vi "smu-dmm-test2.vi"() -> ()   [LabVIEW 2020]
uses:
  Realization/NI DMM/NI DMM.lvclass
  Realization/NI DMM/TypeDefs/DMM waveform settings.ctl
  <instrlib>/niDMM/nidmm.llb/niDMM Waveform Function.ctl
  Realization/NI DMM/TypeDefs/Trigger settings.ctl
  <instrlib>/niDMM/nidmm.llb/niDMM Trigger.ctl
  <instrlib>/niDMM/nidmm.llb/niDMM Slope.ctl
  Realization/PIPX40 Relay/PIPX40 Relay.lvclass
  Realization/PIPX40 Matrix/PIPX40 Matrix.lvclass
  <instrlib>/niDCPower/nidcpower.llb/niDCPower Source Mode.ctl
  <instrlib>/niDCPower/nidcpower.llb/niDCPower Wait For Event - Event.ctl
  <instrlib>/niDCPower/nidcpower.llb/niDCPower Output Function.ctl
panel:
  in  "current limit range":dbl=0.01 format="%.6p"
  in  "voltage level range":dbl=6.0 format="%.6p"
  in  "current limit":dbl=0.01 format="%.6p"
  in  "voltage level":dbl=2.0 format="%.6p"
  in  "Source:Advanced:Source Delay":dbl
  out "Voltage Measurement":dbl
  out "Current Measurement":dbl
  out "Compliance/Limit Reached":bool
  in  "Channel Name":string="0"
  in  "Resource Name":refnum<k15>="NI_SMU1"
  out "relay info":variant
  out "Waveform Graph":dynamicdata(graph)
  out "error out":errorcluster
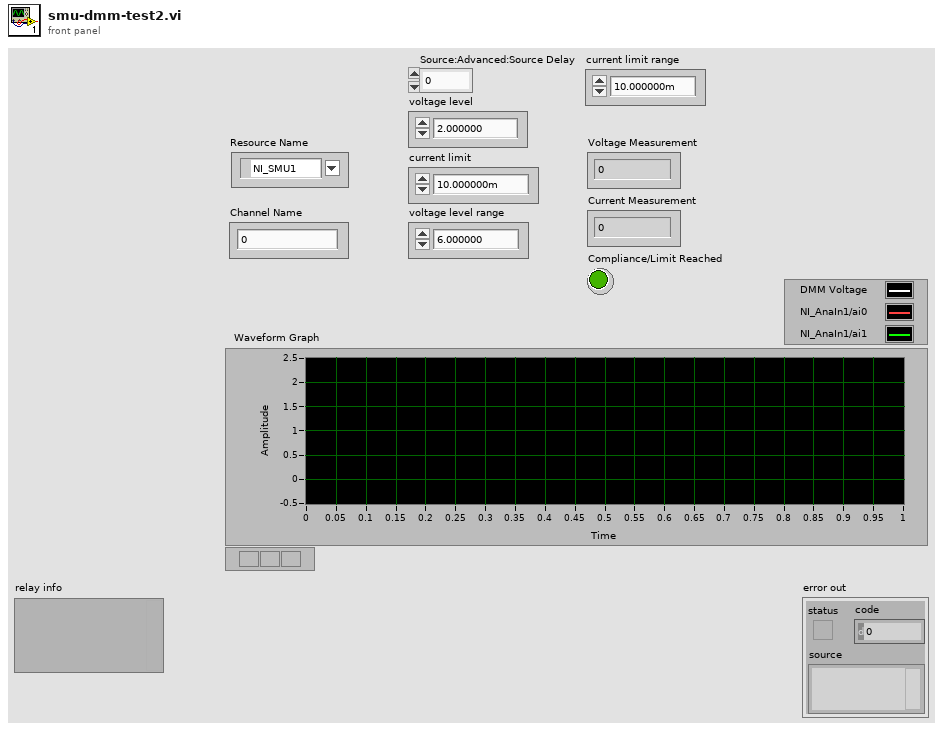
[diagram p1: front panel]
types:
  T1 = typedef "niDCPower Output Function.ctl" = i32
  T2 = typedef "niDCPower Wait For Event - Event.ctl" = i32
  T3 = typedef "niDCPower Source Mode.ctl" = i32
  T4 = typedef "Trigger settings.ctl" = cluster{"Trigger Source":T5, "Trigger Delay (sec)":dbl, "Slope":T6}
  T5 = typedef "niDMM Trigger.ctl" = enum16{"Immediate", "External", "TTL 0", "TTL 1", "TTL 2", "TTL 3", "TTL 4", "TTL 5", "TTL 6", "Software", "TTL 7", "PXI Star", "LBR Trig 1", "Aux Trig 1"}
  T6 = typedef "niDMM Slope.ctl" = enum16{"Rising Edge", "Falling Edge"}
  T7 = typedef "DMM waveform settings.ctl" = cluster{"Waveform Points":i32, "Function":T8, "Rate":dbl, "Range":dbl, "Settle Time":dbl}
  T8 = typedef "niDMM Waveform Function.ctl" = i32
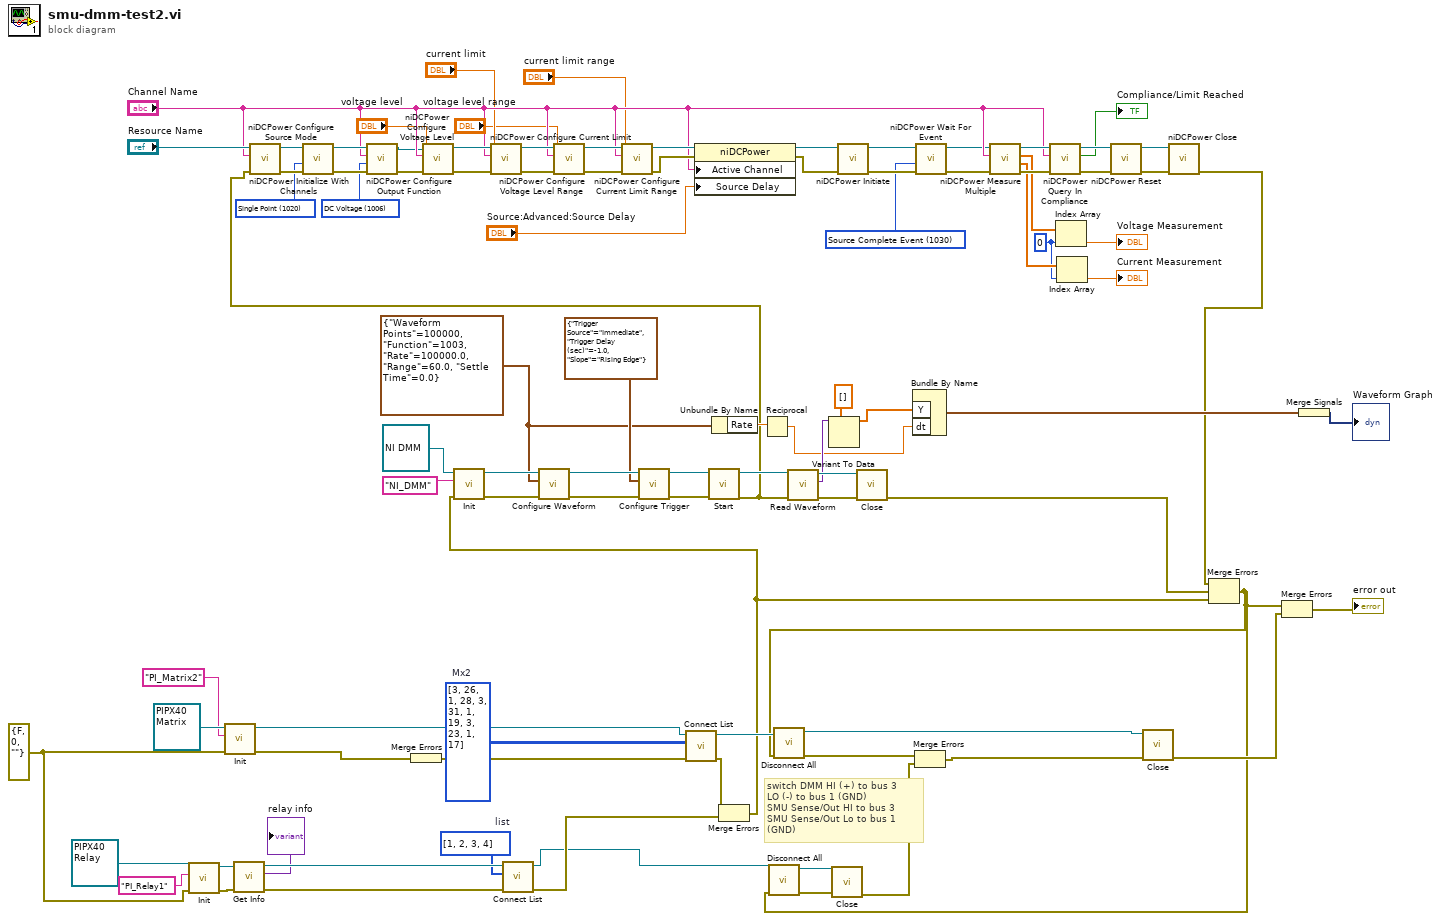
[diagram p0: block diagram]
diagram:
  w8 = T1 1006 items=["DC Voltage"=1006, "DC Current"=1007, "Pulse Voltage"=1049, "Pulse Current"=1050] ("output function")
  w12 = T2 1030 items=["Source Complete Event"=1030, "Measure Complete Event"=1031, "Sequence Iteration Complete Event"=1032, "Sequence Engine Done Event"=1033] ("event")
  w24 = 0 ("index")
  w33 = T3 1020 items=["Single Point"=1020, "Sequence"=1021] ("source mode")
  w55 = i32[] [1, 2, 3, 4]  # list
  w69 = T7 {"Waveform Points"=100000, "Function"=1003, "Rate"=100000.0, "Range"=60.0, "Settle Time"=0.0}
  w54 = errorcluster {"status"=FALSE, "code"=0, "source"=""} ("error in (no error)")
  w93 = i32[][] [[3, 26], [1, 28], [3, 31], [1, 19], [3, 23], [1, 17]]  # Mx2
  # "switch DMM HI (+) to bus 3 \nLO (-) to bus 1 (GND)\nSMU Sense/Out HI to bus 3\nSMU Sense/Out Lo to bus 1 (GND)"
  n1 = call-dynamic "Init.vi"("error in (no error)"=w54, "Params"="PI_Relay1" ("String"), "PIPXI40 Base in"=refnum<class "PIPX40 Relay.lvclass"> refnum ("Pickering.lvlib:PIPX40 Relay.lvclass")) -> ("error out"=w64:errorcluster, "PIPXI40 Base out"=w61:refnum<class "PIPX40 Relay.lvclass">)  [unwired: 7 in]
  n2 = call-dynamic "Init.vi"("error in (no error)"=w54, "Params"="PI_Matrix2" ("String"), "PIPXI40 Base in"=refnum<class "PIPX40 Matrix.lvclass"> refnum ("PIPXI40 Matrix in")) -> ("error out"=w49:errorcluster, "PIPXI40 Base out"=w47:refnum<class "PIPX40 Matrix.lvclass">)  [unwired: 7 in]
  n3 = call-dynamic "Get Info.vi"("error in (no error)"=w64, "PIPXI40 Base in"=w61) -> ("error out"=w58:errorcluster, "Info"=→"relay info":variant, "PIPXI40 Base out"=w60:refnum<class "PIPX40 Relay.lvclass">)  [unwired: 7 in]
  n4 = Merge Errors(w49) -> (w85:errorcluster)
  n5 = call-dynamic "Connect List.vi"("error in (no error)"=w58, "Params"=w55, "PIPXI40 Switching in"=w60) -> ("error out"=w51:errorcluster, "PIPXI40 Switching out"=w50:refnum<class "PIPX40 Relay.lvclass">)  [unwired: 7 in]
  n6 = call-dynamic "Connect List.vi"("error in (no error)"=w85, "Params"=w93, "PIPXI40 Matrix in"=w47) -> ("error out"=w89:errorcluster, "PIPXI40 Matrix out"=w92:refnum<class "PIPX40 Matrix.lvclass">)  [unwired: 7 in]
  n7 = Unbundle By Name(w69) -> ("Rate"=w68:dbl)
  n8 = Merge Errors(w89, w51) -> (w88:errorcluster)
  n9 = call-dynamic "Init.vi"("error in (no error)"=w88, "Params"="NI_DMM", "NI DMM in"=refnum<class "NI DMM.lvclass"> refnum) -> ("error out"=w83:errorcluster, "NI DMM out"=w84:refnum<class "NI DMM.lvclass">)  [unwired: 7 in]
  n10 = call-dynamic "Configure Waveform.vi"("error in (no error)"=w83, "Params"=w69, "NI DMM in"=w84) -> ("error out"=w79:errorcluster, "NI DMM out"=w80:refnum<class "NI DMM.lvclass">)  [unwired: 7 in]
  n11 = call-dynamic "Configure Trigger.vi"("error in (no error)"=w79, "Params"=T4 {"Trigger Source"=enum."Immediate", "Trigger Delay (sec)"=-1.0, "Slope"=enum."Rising Edge"}, "NI DMM in"=w80) -> ("error out"=w77:errorcluster, "NI DMM out"=w78:refnum<class "NI DMM.lvclass">)  [unwired: 7 in]
  n12 = call-dynamic "Start.vi"("error in (no error)"=w77, "DMM in"=w78) -> ("error out"=w7:errorcluster, "DMM out"=w76:refnum<class "NI DMM.lvclass">)  [unwired: 8 in]
  n13 = call <instrlib>:"niDCPower Initialize With Channels.vi"("error in (no error)"=w7, "channels"="Channel Name", "resource name"="Resource Name") -> ("error out"=w37:errorcluster, "instrument handle out"=w36:refnum<k15>)  [unwired: 2 in, 5 out]
  n14 = call <instrlib>:"niDCPower Configure Source Mode.vi"("error in (no error)"=w37, "source mode"=w33, "instrument handle"=w36) -> ("error out"=w35:errorcluster, "instrument handle out"=w34:refnum<k15>)  [unwired: 7 out]
  n15 = call <instrlib>:"niDCPower Configure Output Function.vi"("error in (no error)"=w35, "output function"=w8, "channel name"="Channel Name", "instrument handle"=w34) -> ("error out"=w10:errorcluster, "instrument handle out"=w11:refnum<k15>)  [unwired: 6 out]
  n16 = call <instrlib>:"niDCPower Configure Voltage Level.vi"("error in (no error)"=w10, "voltage level"="voltage level", "channel name"="Channel Name", "instrument handle"=w11) -> ("error out"=w42:errorcluster, "instrument handle out"=w43:refnum<k15>)  [unwired: 6 out]
  n17 = call <instrlib>:"niDCPower Configure Current Limit.vi"("error in (no error)"=w42, "current limit"="current limit", "channel name"="Channel Name", "instrument handle"=w43) -> ("error out"=w32:errorcluster, "instrument handle out"=w31:refnum<k15>)  [unwired: 1 in, 5 out]
  n18 = call <instrlib>:"niDCPower Configure Voltage Level Range.vi"("error in (no error)"=w32, "voltage level range"="voltage level range", "channel name"="Channel Name", "instrument handle"=w31) -> ("error out"=w30:errorcluster, "instrument handle out"=w29:refnum<k15>)  [unwired: 6 out]
  n19 = call <instrlib>:"niDCPower Configure Current Limit Range.vi"("error in (no error)"=w30, "current limit range"="current limit range", "channel name"="Channel Name", "instrument handle"=w29) -> ("error out"=w18:errorcluster, "instrument handle out"=w21:refnum<k15>)  [unwired: 6 out]
  n20 = property class="niDCPower"(reference=w21, error in=w18, "Active Channel"="Channel Name", "Source Delay"="Source:Advanced:Source Delay") -> (reference out=w20:refnum<k15>, error out=w19:errorcluster)
  n21 = Reciprocal(x=w68) -> (1/x=w67:dbl)
  n22 = call-dynamic "Read Waveform.vi"("error in (no error)"=w7, "NI DMM in"=w76) -> ("error out"=w74:errorcluster, "Data"=w72:variant, "NI DMM out"=w73:refnum<class "NI DMM.lvclass">)  [unwired: 7 in]
  n23 = Variant To Data(type=dbl[] [], Variant=w72) -> (data=w70:dbl[])  [unwired: 1 in, 1 out]
  n24 = call <instrlib>:"niDCPower Initiate.vi"("error in (no error)"=w19, "instrument handle"=w20) -> ("error out"=w14:errorcluster, "instrument handle out"=w16:refnum<k15>)  [unwired: 2 in, 6 out]
  n25 = call-dynamic "Close.vi"("error in (no error)"=w74, "NI DMM in"=w73) -> ("error out"=w65:errorcluster)  [unwired: 8 in, 1 out]
  n26 = Bundle By Name("Y"=w70, "dt"=w67) -> (w66:waveform(dbl))  [unwired: 1 in]
  n27 = call <instrlib>:"niDCPower Wait For Event.vi"("error in (no error)"=w14, "event"=w12, "instrument handle"=w16) -> ("error out"=w13:errorcluster, "instrument handle out"=w15:refnum<k15>)  [unwired: 1 in, 6 out]
  n28 = call <instrlib>:"niDCPower Measure Multiple.vi"("error in (no error)"=w13, "channel name"="Channel Name", "instrument handle"=w15) -> ("error out"=w27:errorcluster, "current measurements"=w25:dbl[], "voltage measurements"=w26:dbl[], "instrument handle out"=w28:refnum<k15>)  [unwired: 5 out]
  n29 = call <instrlib>:"niDCPower Query In Compliance.vi"("error in (no error)"=w27, "channel name"="Channel Name", "instrument handle"=w28) -> ("error out"=w38:errorcluster, "in compliance?"=→"Compliance/Limit Reached":bool, "instrument handle out"=w41:refnum<k15>)  [unwired: 6 out]
  n30 = Index Array(array=w26, index=w24) -> (element=→"Voltage Measurement":dbl)
  n31 = Index Array(array=w25, index=w24) -> (element=→"Current Measurement":dbl)
  n32 = call <instrlib>:"niDCPower Reset.vi"("error in (no error)"=w38, "instrument handle"=w41) -> ("error out"=w39:errorcluster, "instrument handle out"=w40:refnum<k15>)  [unwired: 2 in, 6 out]
  n33 = call <instrlib>:"niDCPower Close.vi"("error in (no error)"=w39, "instrument handle"=w40) -> ("error out"=w6:errorcluster)  [unwired: 9 out]
  n34 = Merge Errors(w6, w65, w88) -> (w53:errorcluster)
  n35 = call-dynamic "Disconnect All.vi"("error in (no error)"=w53, "PIPXI40 Switching in"=w50) -> ("error out"=w56:errorcluster, "PIPXI40 Switching out"=w57:refnum<class "PIPX40 Relay.lvclass">)  [unwired: 8 in]
  n36 = call-dynamic "Disconnect All.vi"("error in (no error)"=w53, "PIPXI40 Matrix in"=w92) -> ("error out"=w91:errorcluster, "PIPXI40 Matrix out"=w45:refnum<class "PIPX40 Matrix.lvclass">)  [unwired: 8 in]
  n37 = call-dynamic "Close.vi"("error in (no error)"=w56, "PIPXI40 Base in"=w57) -> ("error out"=w52:errorcluster)  [unwired: 8 in, 1 out]
  n38 = Merge Errors(w91, w52) -> (w90:errorcluster)
  n39 = call-dynamic "Close.vi"("error in (no error)"=w90, "PIPXI40 Base in"=w45) -> ("error out"=w87:errorcluster)  [unwired: 8 in, 1 out]
  n40 = Merge Errors(w53, w87) -> (→"error out":errorcluster)
  n41 = Merge Signals(w66) -> (→"Waveform Graph":dynamicdata)
